vi "Gripper Control Loop CAN.vi"(8 "error in":errorcluster) -> ()   [LabVIEW 2014, in "Elevator System.lvlib"]
uses:
  Elevator System.lvlib
  <vilib>/Rock Robotics/WPI/MotorControl/WPI_MotorControlDeviceRef.ctl
  <vilib>/Rock Robotics/WPI/MotorControl/WPI_MotorControlType.ctl
  <vilib>/Rock Robotics/SystemInterfaces/Typedef/FPGA_TypedefDigitalModule.ctl
  <vilib>/Rock Robotics/SystemInterfaces/DIO/FPGA_DIOPWMChannel.ctl
  <vilib>/Rock Robotics/WPI/PWM/WPI_PWMDeadband.ctl
  <vilib>/Rock Robotics/WPI/CAN/Jaguar/SubVIs/WPI_CANJaguar_ControlMode.ctl
  <vilib>/Rock Robotics/WPI/CAN/TalonSRX/WPI_CANTalonSRX_APIControlMode.ctl
  <vilib>/Rock Robotics/WPI/PWM/WPI_PWMTransform_ConPane.ctl
  Typedef/GripperNotifierType.ctl
  Public/Sensors Global.vi
panel:
  out "Right":dbl(graph)
  out "Left":dbl(graph)
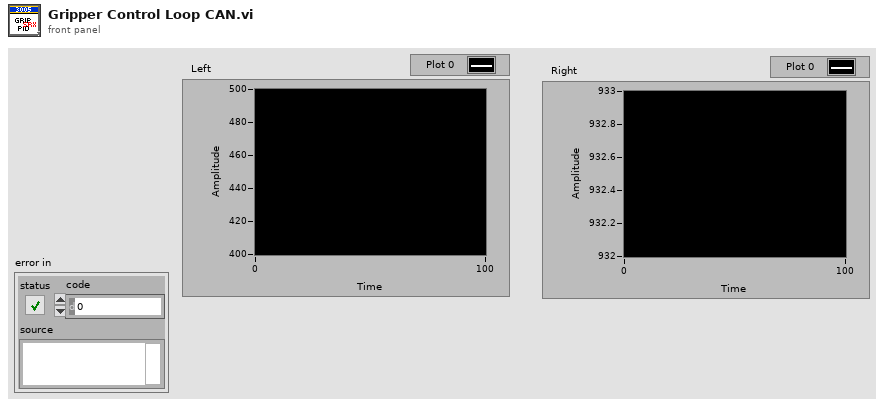
[diagram p1: front panel]
types:
  T1 = typedef "WPI_MotorControlDeviceRef.ctl" = cluster{"DeviceStatus":errorcluster, "Type":T2, "PWM":cluster{"Controller":T3, "PWM Channel":T4, "DeadBand":T5}, "CAN":cluster{"Device Number":u8, "Control Mode":T6, "Semaphore":T7, "Max Vout":dbl, "TalonSRX Control Mode":T8}, "Invert":bool, "TransformRef":T9, "InvTransformRef":T9}
  T2 = typedef "WPI_MotorControlType.ctl" = enum16{"PWM", "CAN", "CANTalonSRX"}
  T3 = typedef "FPGA_TypedefDigitalModule.ctl" = enum16{"Controller 1"}
  T4 = typedef "FPGA_DIOPWMChannel.ctl" = enum8{"PWM 0", "PWM 1", "PWM 2", "PWM 3", "PWM 4", "PWM 5", "PWM 6", "PWM 7", "PWM 8", "PWM 9", "PWM MXP 0", "PWM MXP 1", "PWM MXP 2", "PWM MXP 3", "PWM MXP 4", "PWM MXP 5", "PWM MXP 6", "PWM MXP 7", "PWM MXP 8", "PWM MXP 9", "Invalid"}
  T5 = typedef "WPI_PWMDeadband.ctl" = cluster{"Name":string, "maxPositivePwm":i32, "minPositivePwm":i32, "centerPwm":i32, "maxNegativePwm":i32, "minNegativePwm":i32, "angularRange":u16}
  T6 = typedef "WPI_CANJaguar_ControlMode.ctl" = enum8{"Percent VBus", "Current", "Speed", "Position", "Voltage"}
  T7 = typedef "Semaphore RefNum" = refnum<k1>
  T8 = typedef "WPI_CANTalonSRX_APIControlMode.ctl" = enum8{"Percent VBus", "Speed", "Position", "Slave", "Unchanged / Invalid"}
  T9 = typedef "WPI_PWMTransform_ConPane.ctl" = refnum<vi>
  T10 = typedef "Elevator System.lvlib/GripperNotifierType.ctl" = cluster{"SP Left":dbl, "SP Right":dbl}
  T11 = cluster{"Output":dbl, "GripperMotorL":T1, "GripperMotorR":T1, "notifier":refnum<notifier>, "Setpoint":T10}
  T12 = typedef "GripperNotifierType.ctl" = cluster{"SP Left":dbl, "SP Right":dbl}
  T13 = typedef "WPI_CANTalonSRX_GlobalStatus.ctl" = cluster{"Applied Throttle":dbl, "Module Enabled":bool, "CAN Error":errorcluster, "Closed Loop Error":dbl, "Forward Limit Switch Closed":bool, "Reverse Limit Switch Closed":bool, "Sensor Position":dbl, "Sensor Velocity":dbl, "Current":dbl, "Sticky Fault - Over Temp":bool, "Sticky Fault - Under Voltage":bool, "Sticky Fault - Forward Limit":bool, "Sticky Fault - Reverse Limit":bool, "Sticky Fault - Forward Soft Limit":bool, "Sticky Fault - Reverse Soft Limit":bool, "Brake is Enabled":bool, "Encoder Position":dbl, "Encoder Velocity":dbl, "Encoder Index Count":dbl, "Encoder A Pin State":bool, "Encoder B Pin State":bool, "Encoder Index Pin State":bool, "Analog In":dbl, "Analog In Velocity":dbl, "Temperature (C)":dbl, "Battery Voltage":dbl}
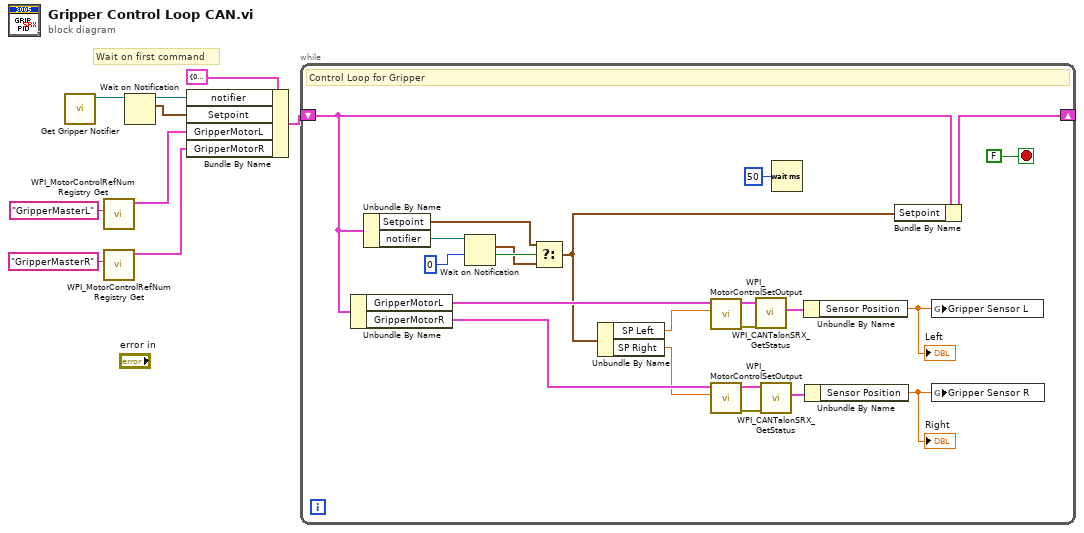
[diagram p0: block diagram]
diagram:
  # "Wait on first command"
  n1 = call "Get Gripper Notifier.vi"() -> ("Notifier out"=w7:refnum<notifier>)  [unwired: 11 in]
  n2 = call <vilib>:"WPI_MotorControlRefNum Registry Get.vi"("refnum name"="GripperMasterL") -> ("MotorControlDevRef"=w3:T1)  [unwired: 9 in, 1 out]
  n3 = call <vilib>:"WPI_MotorControlRefNum Registry Get.vi"("refnum name"="GripperMasterR") -> ("MotorControlDevRef"=w6:T1)  [unwired: 9 in, 1 out]
  n4 = Wait on Notification(notifier=w7) -> (notifier out=w2:refnum<notifier>, notification=w1:T12)  [unwired: 3 in, 2 out]
  n5 = Bundle By Name(cluster=T11 {"Output"=0.0, "GripperMotorL"={"DeviceStatus"={"status"=FALSE, "code"=0, "source"=""}, "Type"=enum."PWM", "PWM"={"Controller"=enum."Controller 1", "PWM Channel"=enum."Invalid", "DeadBand"={"Name"="", "maxPositivePwm"=0, "minPositivePwm"=0, "centerPwm"=0, "maxNegativePwm"=0, "minNegativePwm"=0, "angularRange"=0}}, "CAN"={"Device Number"=0, "Control Mode"=enum."Percent VBus", "Semaphore"=refnum, "Max Vout"=12.0, "TalonSRX Control Mode"=enum."Percent VBus"}, "Invert"=FALSE, "TransformRef"=refnum, "InvTransformRef"=refnum}, "GripperMotorR"={"DeviceStatus"={"status"=FALSE, "code"=0, "source"=""}, "Type"=enum."PWM", "PWM"={"Controller"=enum."Controller 1", "PWM Channel"=enum."Invalid", "DeadBand"={"Name"="", "maxPositivePwm"=0, "minPositivePwm"=0, "centerPwm"=0, "maxNegativePwm"=0, "minNegativePwm"=0, "angularRange"=0}}, "CAN"={"Device Number"=0, "Control Mode"=enum."Percent VBus", "Semaphore"=refnum, "Max Vout"=12.0, "TalonSRX Control Mode"=enum."Percent VBus"}, "Invert"=FALSE, "TransformRef"=refnum, "InvTransformRef"=refnum}, "notifier"=refnum, "Setpoint"={"SP Left"=0.0, "SP Right"=0.0}}, "notifier"=w2, "Setpoint"=w1, "GripperMotorL"=w3, "GripperMotorR"=w6) -> (w8:T11)
  n6 = while {
    shift-right: [w22] -> _
    shift-left: w8 -> [w23]
    stop <- FALSE stop-if-true
    # "Control Loop for Gripper"
    n7 = Unbundle By Name(w23) -> ("GripperMotorL"=w29:T1, "GripperMotorR"=w28:T1)
    n8 = Unbundle By Name(w23) -> ("Setpoint"=w19:T10, "notifier"=w30:refnum<notifier>)
    n9 = Wait on Notification(notifier=w30, timeout in ms (-1)=0) -> (notification=w20:T10, timed out?=w21:bool)  [unwired: 2 in, 2 out]
    n10 = Select(t=w19, s=w21, f=w20) -> (s? t:f=w12:T10)
    n11 = Unbundle By Name(w12) -> ("SP Left"=w11:dbl, "SP Right"=w10:dbl)
    n12 = call <vilib>:"WPI_MotorControlSetOutput.vi"("Output"=w11, "MotorControlDevRef"=w29) -> ("error out"=w17:errorcluster, "MotorControlDevRef"=w16:T1)  [unwired: 7 in, 1 out]
    n13 = call <vilib>:"WPI_MotorControlSetOutput.vi"("Output"=w10, "MotorControlDevRef"=w28) -> ("error out"=w26:errorcluster, "MotorControlDevRef"=w25:T1)  [unwired: 7 in, 1 out]
    n14 = call <vilib>:"WPI_CANTalonSRX_GetStatus.vi"("error in (no error)"=w17, "CAN Talon SRX Ref"=w16) -> ("Talon SRX Status"=w15:T13)  [unwired: 7 in, 2 out]
    n15 = call <vilib>:"WPI_CANTalonSRX_GetStatus.vi"("error in (no error)"=w26, "CAN Talon SRX Ref"=w25) -> ("Talon SRX Status"=w24:T13)  [unwired: 7 in, 2 out]
    n16 = Wait (ms)(milliseconds to wait=u32 50) -> ()  [unwired: 1 out]
    n17 = Unbundle By Name(w15) -> ("Sensor Position"=w13:dbl)
    "Left" <- w13
    n18 = Unbundle By Name(w24) -> ("Sensor Position"=w14:dbl)
    "Right" <- w14
    n19 = Bundle By Name(cluster=w23, "Setpoint"=w12) -> (w22:T11)
    n20 = global write "Sensors Global.vi" "Gripper Sensor L"(w13) -> ()
    n21 = global write "Sensors Global.vi" "Gripper Sensor R"(w14) -> ()
  }
